vi "Lookup Child by Name.vi"(8 "error in (no error)":errorcluster, 10 "Name":string, 11 "Seq Element in":refnum<class "Seq Element.lvclass">) -> (0 "error out":errorcluster, 3 "Seq Element out":refnum<class "Seq Element.lvclass">)   [LabVIEW 2020, in "Seq Element.lvclass"]
uses:
  Seq Element.lvclass
  Seq Element.lvclass/Seq Element.ctl
  lv-cdm/CDM-Config/Config Element/Config Element.lvclass
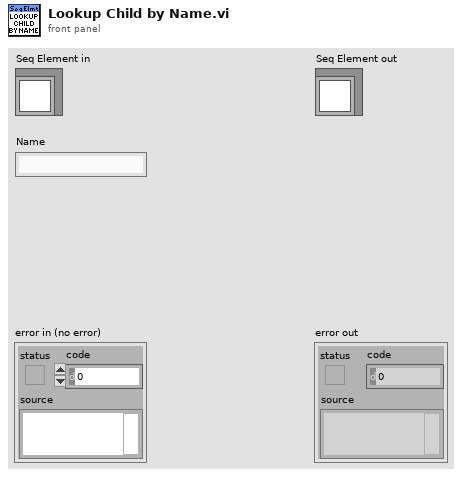
[diagram p1: front panel]
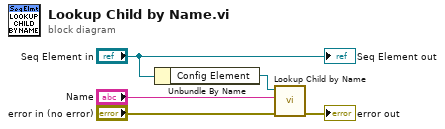
[diagram p0: block diagram]
diagram:
  n1 = Unbundle By Name("Seq Element in") -> ("Config Element"=w4:refnum<class "Config Element.lvclass">)
  n2 = call "Lookup Child by Name.vi"("error in (no error)"="error in (no error)", "Name"="Name", "Config Element in"=w4) -> ("error out"=→"error out":errorcluster)  [unwired: 5 in, 3 out]
  "Seq Element out" <- "Seq Element in"
